vi "unused_toBoolUE.vi"(8 "error in":errorcluster, 11 "ITaskChannel":refnum<class "ITaskChannel.lvclass">) -> (0 "error out":errorcluster, 3 "userEventRef":refnum<user-event>)   [LabVIEW 2023]
uses:
  ITaskChannel/ITaskChannel.lvclass
  BoolUETaskChannel/BoolUETaskChannel.lvclass
  BoolUserEventStopMech/Read userEventRef.vi
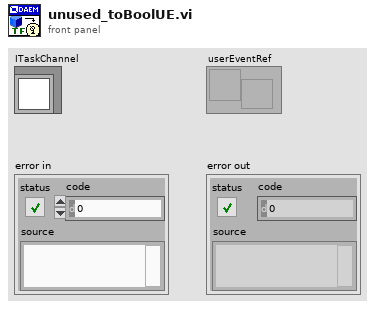
[diagram p1: front panel]
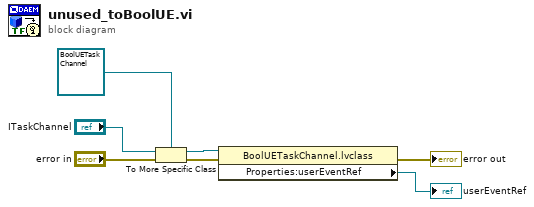
[diagram p0: block diagram]
diagram:
  n1 = To More Specific Class(target class=refnum<class "BoolUETaskChannel.lvclass"> refnum ("TLC_Daemon.lvlib:BoolUETaskChannel.lvclass"), reference="ITaskChannel", error in="error in") -> (specific class reference=w5:refnum<class "BoolUETaskChannel.lvclass">, error out=w6:errorcluster)
  n2 = property class="BoolUETaskChannel.lvclass"(reference=w5, error in=w6) -> (error out=→"error out":errorcluster, "Properties:userEventRef"=→"userEventRef":refnum<user-event>)  [unwired: 1 out]
